vi "lab-task2-JanntAllahSabry.vi"() -> ()   [LabVIEW 2020]
uses:
  <vilib>/Utility/file.llb/Write Delimited Spreadsheet (string).vi
  <vilib>/picture/3D Picture Control/Object/Add Object (no reference).vi
  <vilib>/picture/3D Picture Control/Object/Create Object (name).vi
  <vilib>/Instr/_visa.llb/VISA Configure Serial Port (Instr).vi
  <vilib>/picture/3D Picture Control/NI_3D Picture Control.lvlib
panel:
  in  "test":string
  in  "stop":bool
  in  "file path (dialog if empty)":path
  out "mpu (x,y,z) Chart":T1(graph)
  out "z":dbl(slide) scale=-10.0..10.0
  out "y":dbl(slide) scale=-10.0..10.0
  out "x":dbl(slide) scale=-10.0..10.0
  out "3D Picture":refnum<vi>(3d-picture)
  out "PRESSURE":dbl
  out "Altitude & Pressure":T1(graph)
  out "ALTITUDE":dbl
  out "RH":dbl
  out "RH & Temp chart":T1(graph)
  out "Temp":dbl
  in  "VISA resource name":refnum<visa-resource-name>
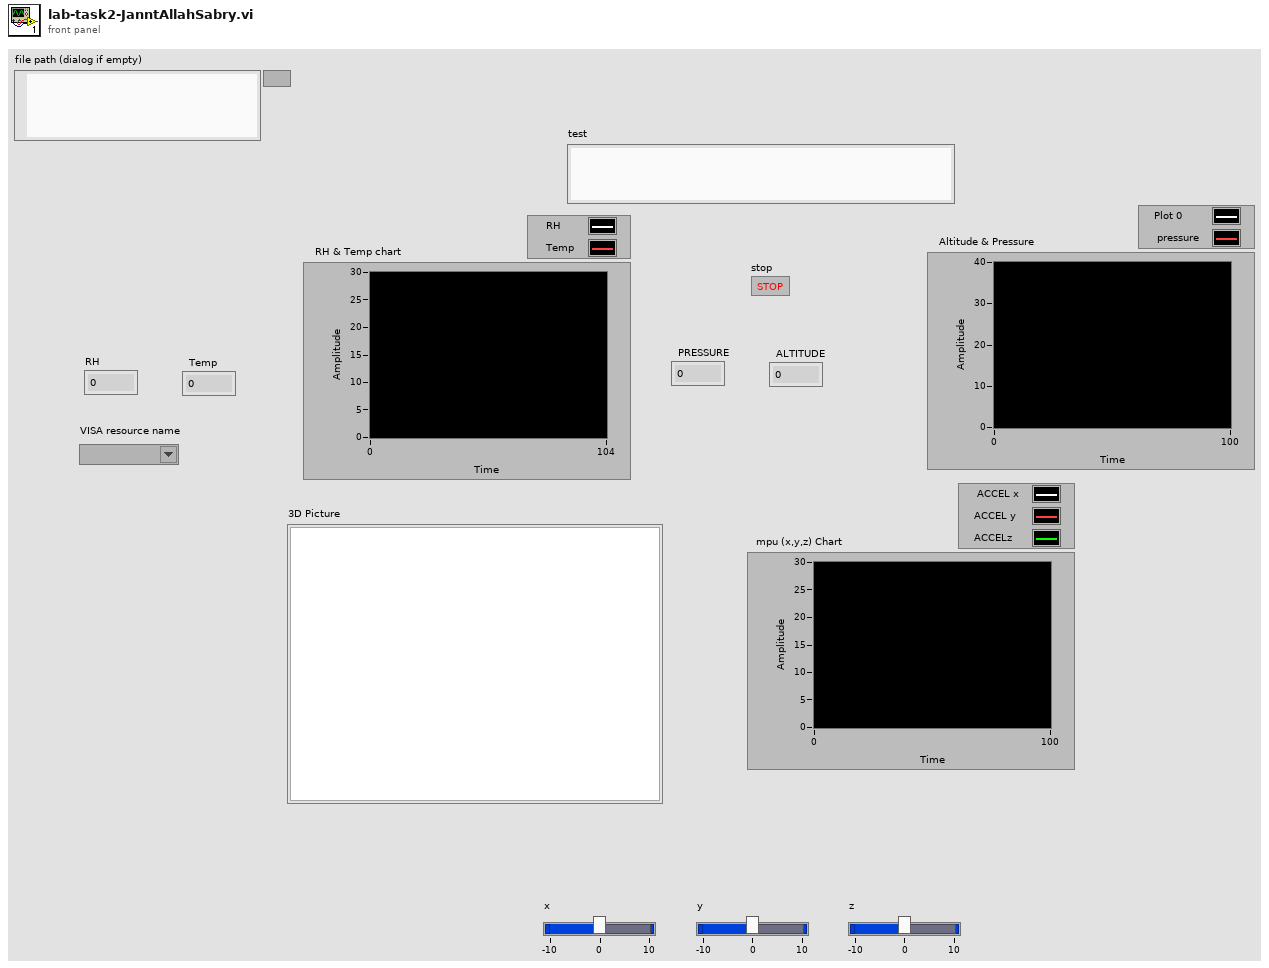
[diagram p1: front panel]
types:
  T1 = cluster{"[0]":dbl, "[1]":dbl, "[2]":dbl, "[3]":dbl, "[4]":dbl, "[5]":dbl, "[6]":dbl, "[7]":dbl, "[8]":dbl}
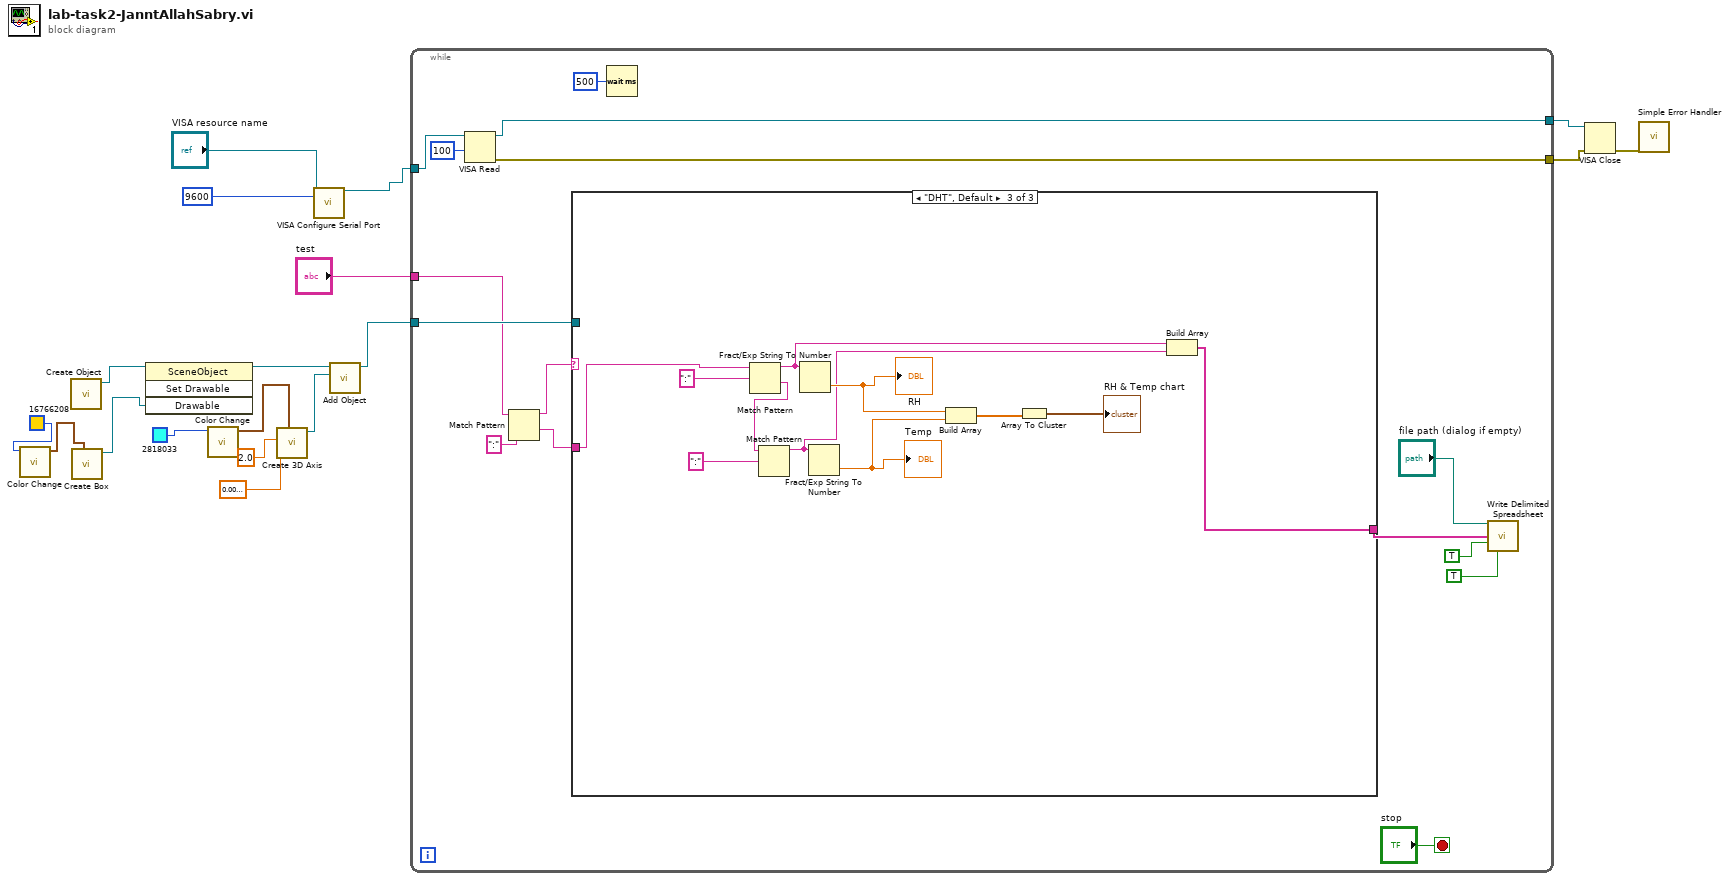
[diagram p0: block diagram]
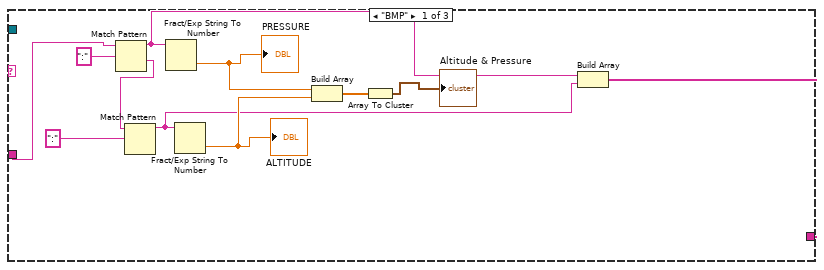
[diagram p2: hidden frame]
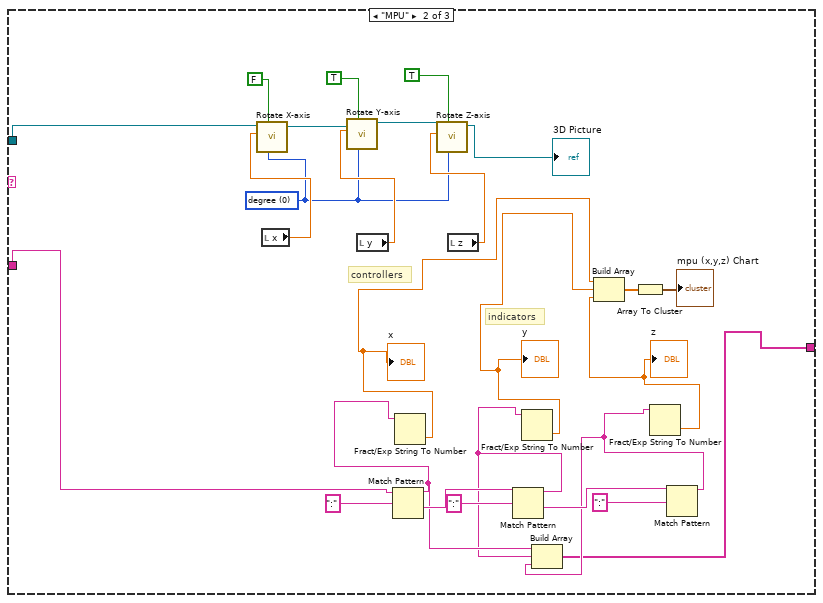
[diagram p3: hidden frame]
diagram:
  n1 = call <vilib>:"Color Change.vi"("Color"=u32 16766208 ("Color Box")) -> ("RGBA"=w15:cluster{"R":sgl, "G":sgl, "B":sgl, "A":sgl})  [unwired: 10 in]
  n2 = call-poly <vilib>:"Create Object.vi"() -> ("Scene:New Object"=w18:refnum<vi>)  [unwired: 10 in, 1 out]
  n3 = call <vilib>:"Create Box.vi"("Color"=w15) -> ("New Box Refnum"=w17:refnum<vi>)  [unwired: 9 in, 1 out]
  n4 = invoke class="SceneObject" method="Set Drawable"(reference=w18, "Drawable"=w17) -> (reference out=w14:refnum<vi>)  [unwired: 2 in, 3 out]
  n5 = call <vilib>:"Color Change.vi"("Color"=u32 2818033 ("Color Box")) -> ("RGBA"=w11:cluster{"R":sgl, "G":sgl, "B":sgl, "A":sgl})  [unwired: 10 in]
  n6 = call <vilib>:"Create 3D Axis.vi"("Color"=w11, "Radius"=sgl 0.01, "Length"=sgl 2.0) -> ("New Object Refnum"=w13:refnum<vi>)  [unwired: 7 in, 1 out]
  n7 = call-poly "VISA Configure Serial Port"("VISA resource name"="VISA resource name", "baud rate (9600)"=u32 9600) -> ("VISA resource name out"=w5:refnum<visa-resource-name>)  [unwired: 12 in, 1 out]
  n8 = call-poly <vilib>:"Add Object.vi"("New Object In"=w13, "Scene Object In"=w14) -> ("Scene Object Out"=w8:refnum<vi>)  [unwired: 8 in, 1 out]
  n9 = while {
    tunnel: w8 -> [w31]
    tunnel: w5 -> [w23]
    tunnel: [w22] -> w3
    tunnel: [w21] -> w2
    tunnel: "test" -> [w19]
    stop <- "stop" stop-if-true
    n10 = VISA Read(VISA resource name=w23, byte count=u32 100) -> (VISA resource name out=w22:refnum<visa-resource-name>, error out=w21:errorcluster)  [unwired: 1 in, 2 out]
    n11 = Match Pattern(string=w19, regular expression=":") -> (before substring=w30:string, after substring=w32:string)  [unwired: 1 in, 2 out]
    n12 = case shown="\"DHT\", Default" w30 {
      tunnel: w32 -> [w34 w45 w71]
      tunnel: w31 -> [_ w52 _]
      tunnel: [w37 w48 w74] -> w27
      frame "BMP" {
        n13 = Match Pattern(string=w34, regular expression=":") -> (before substring=w39:string, after substring=w42:string)  [unwired: 1 in, 2 out]
        n14 = Match Pattern(string=w42, regular expression=":") -> (before substring=w38:string)  [unwired: 1 in, 3 out]
        n15 = Fract/Exp String To Number(string=w39) -> (number=w43:dbl)  [unwired: 3 in, 1 out]
        "PRESSURE" <- w43
        n16 = Fract/Exp String To Number(string=w38) -> (number=w44:dbl)  [unwired: 3 in, 1 out]
        "ALTITUDE" <- w44
        n17 = Build Array(w43, w44) -> (w36:dbl[])
        n18 = Array To Cluster(array=w36) -> (cluster=→"Altitude & Pressure":T1)
        n19 = Build Array(w39, w38) -> (w37:string[])
      }
      frame "MPU" {
        w56 = u16 0 items=["degree", "radians"] ("angle unit")
        # "indicators"
        # "controllers"
        n20 = local read "x"() -> (w63:dbl)
        n21 = call <vilib>:"Rotate X-axis.vi"("angle unit"=w56, "Relative?"=FALSE, "angle"=w63, "Scene Object In"=w52) -> ("Scene Object Out"=w60:refnum<vi>)  [unwired: 6 in, 1 out]
        n22 = local read "y"() -> (w64:dbl)
        n23 = call <vilib>:"Rotate Y-axis.vi"("angle unit"=w56, "Relative?"=TRUE, "angle"=w64, "Scene Object In"=w60) -> ("Scene Object Out"=w61:refnum<vi>)  [unwired: 6 in, 1 out]
        n24 = Match Pattern(string=w45, regular expression=":") -> (before substring=w51:string, after substring=w67:string)  [unwired: 1 in, 2 out]
        n25 = Fract/Exp String To Number(string=w51) -> (number=w68:dbl)  [unwired: 3 in, 1 out]
        "x" <- w68
        n26 = local read "z"() -> (w65:dbl)
        n27 = call <vilib>:"Rotate Z-axis.vi"("angle unit"=w56, "Relative?"=TRUE, "angle"=w65, "Scene Object In"=w61) -> ("Scene Object Out"=→"3D Picture":refnum<vi>)  [unwired: 6 in, 1 out]
        n28 = Match Pattern(string=w67, regular expression=":") -> (before substring=w50:string, after substring=w66:string)  [unwired: 1 in, 2 out]
        n29 = Fract/Exp String To Number(string=w50) -> (number=w69:dbl)  [unwired: 3 in, 1 out]
        "y" <- w69
        n30 = Match Pattern(string=w66, regular expression=":") -> (before substring=w49:string)  [unwired: 1 in, 3 out]
        n31 = Build Array(w51, w50, w49) -> (w48:string[])
        n32 = Fract/Exp String To Number(string=w49) -> (number=w70:dbl)  [unwired: 3 in, 1 out]
        "z" <- w70
        n33 = Build Array(w68, w69, w70) -> (w47:dbl[])
        n34 = Array To Cluster(array=w47) -> (cluster=→"mpu (x,y,z) Chart":T1)
      }
      frame "DHT", Default {
        n35 = Match Pattern(string=w71, regular expression=":") -> (before substring=w76:string, after substring=w79:string)  [unwired: 1 in, 2 out]
        n36 = Match Pattern(string=w79, regular expression=":") -> (before substring=w75:string)  [unwired: 1 in, 3 out]
        n37 = Fract/Exp String To Number(string=w76) -> (number=w80:dbl)  [unwired: 3 in, 1 out]
        "RH" <- w80
        n38 = Fract/Exp String To Number(string=w75) -> (number=w81:dbl)  [unwired: 3 in, 1 out]
        "Temp" <- w81
        n39 = Build Array(w80, w81) -> (w73:dbl[])
        n40 = Array To Cluster(array=w73) -> (cluster=→"RH & Temp chart":T1)
        n41 = Build Array(w76, w75) -> (w74:string[])
      }
    }
    n42 = Wait (ms)(milliseconds to wait=u32 500) -> ()  [unwired: 1 out]
    n43 = call-poly <vilib>:"Write Delimited Spreadsheet.vi"("file path (dialog if empty)"="file path (dialog if empty)", "1D data"=w27, "append to file? (new file:F)"=TRUE, "transpose? (no:F)"=TRUE) -> ()  [unwired: 10 in, 2 out]
  }
  n44 = VISA Close(VISA resource name=w3, error in (no error)=w2) -> (error out=w4:errorcluster)
  n45 = call <vilib>:"Simple Error Handler.vi"("error in (no error)"=w4) -> ()  [unwired: 4 in, 5 out]
